vi "Read Plugin Locaiton on Disk.vi"(8 "error in (no error)":errorcluster, 11 "Plugin Handler Initialize in":refnum<class "Plugin Handler Initialize.lvclass">) -> (0 "error out":errorcluster, 2 "Plugin Locaiton on Disk":path, 3 "Plugin Handler Initialize out":refnum<class "Plugin Handler Initialize.lvclass">)   [LabVIEW 2011, in "Plugin Handler Initialize.lvclass"]
uses:
  Plugin Handler Initialize.lvclass
  Plugin Handler Initialize.lvclass/Plugin Handler Initialize.ctl
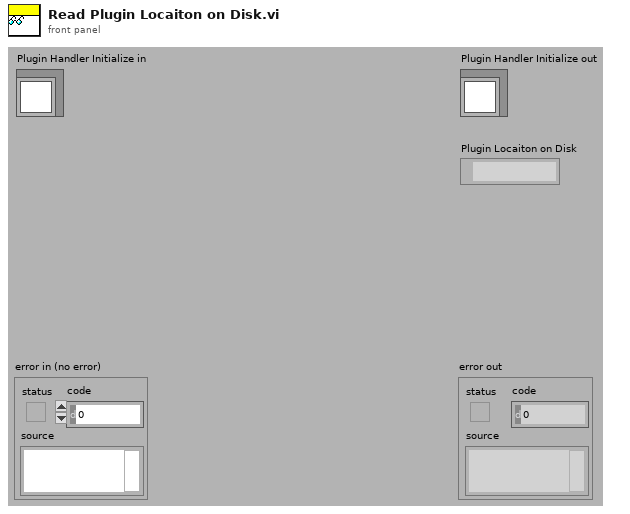
[diagram p1: front panel]
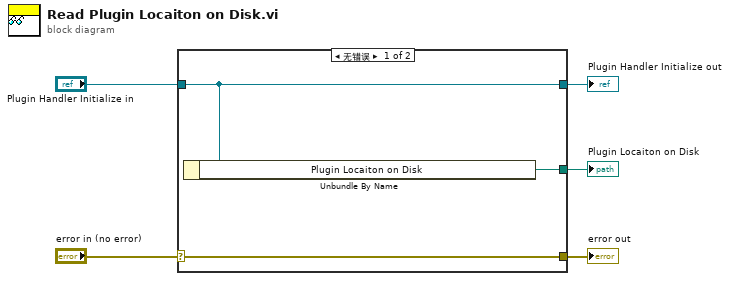
[diagram p0: block diagram]
diagram:
  n1 = case shown="无错误" "error in (no error)" {
    selector: "error in (no error)" -> [w8 w9]
    tunnel: [w8 w9] -> w4
    tunnel: [w7 w10] -> w2
    tunnel: "Plugin Handler Initialize in" -> [w7 w10]
    tunnel: [w6 _] -> w1
    frame No Error {
      n2 = Unbundle By Name(w7) -> ("Plugin Locaiton on Disk"=w6:path)
    }
    frame Error {
    }
  }
  "error out" <- w4
  "Plugin Handler Initialize out" <- w2
  "Plugin Locaiton on Disk" <- w1
